vi "Test_API_GetGlobalLogInstance_ValidLogInstanceReturned.vi"(8 "error in (no error)":errorcluster, 11 "TestCase in":refnum<class "TestComposedLog.lvclass">) -> (0 "error out":errorcluster, 3 "TestCase out":refnum<class "TestComposedLog.lvclass">)   [LabVIEW 2017, in "TestComposedLog.lvclass"]
uses:
  TestComposedLog.lvclass
  Source/Composed Log/Types/Log Level.ctl
  Source/Composed Log/LoggerReference/LoggerReference.lvclass/LoggerReference.ctl
  26ac907e-b197-4f92-b50b-edca335a3ee8.vi
  26ac907e-b197-4f92-b50b-edca335a3ee8.vi/98f69271-1de1-4081-8ac1-8b840b0807ac.vi
  Source/Composed Log/Singleton Event Log/Get Nested Global Log Instance.vi/b2f05d58-65df-4e80-8f90-78513ac31376.vi
  Source/Composed Log/LoggerReference/Return Aggregate Queues.vi
  Source/Composed Log/LoggerReference/Add Aggregate Log.vi
  26ac907e-b197-4f92-b50b-edca335a3ee8.vi/98f69271-1de1-4081-8ac1-8b840b0807ac.vi/bbd2f978-e444-4445-9202-4eeb40a61ae4.vi
  Source/Composed Log/Singleton Event Log/Get Nested Global Log Instance.vi/b2f05d58-65df-4e80-8f90-78513ac31376.vi/e1ecde32-be62-4caa-aa7a-1c02d969ae2d.vi
  Source/Composed Log/LoggerReference/Send Add Sink.vi
  Source/LVQueue Sink/LVQueue Sink.lvclass
  C:/CS/Internal/LabVIEW/Logger/Source/Composed Log/Log Sink/Log Sink.lvclass
  Source/Composed Log/Application Logger/Launch Worker Loop.vi
  Source/Composed Log/LoggerReference/Initialize Logger Instance.vi
  Source/Composed Log/Singleton Event Log/Logger Queue FGV.vi
  Source/Composed Log/Singleton Event Log/Shared Instance FGV.vi
  Source/Composed Log/IErrorFormat/IErrorFormat.lvclass
  Source/Composed Log/LoggerReference/LoggerReference.lvclass
  Source/Composed Log/Log Sink/Log Sink.lvclass
  <vilib>/addons/_JKI Toolkits/VI Tester/TestCase.llb/TestCase.lvclass
  Source/Composed Log/Composed Log.lvlib
  Source/Composed Log/Singleton Event Log/Singleton Event Log.lvlib
  C:/Program Files (x86)/National Instruments/LabVIEW 2017/vi.lib/addons/_JKI Toolkits/VI Tester/TestCase.llb/TestCase.lvclass
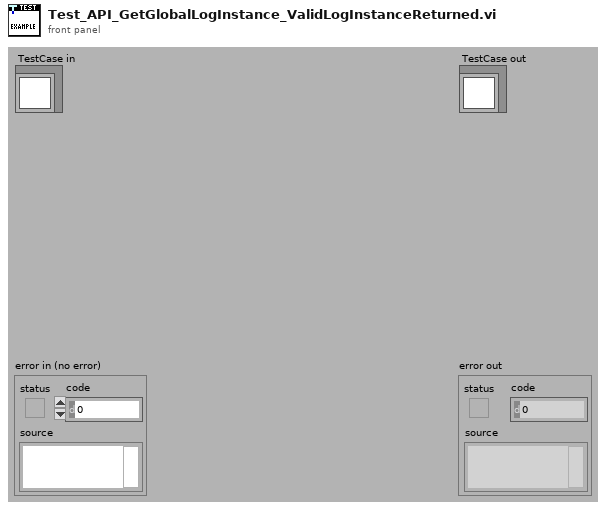
[diagram p1: front panel]
types:
  T1 = typedef "Composed Log.lvlib/Log Level.ctl" = enum16{"Debug", "Info", "Warning", "Error", "Critical"}
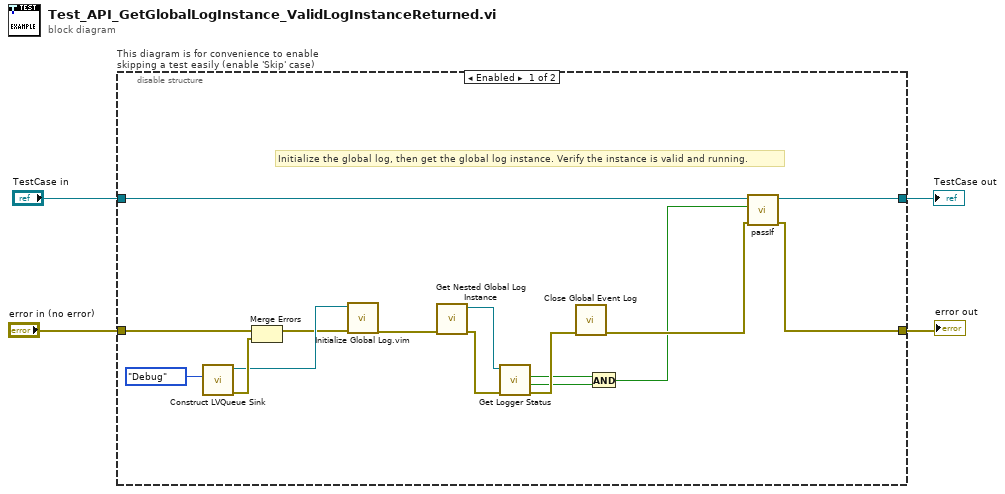
[diagram p0: block diagram]
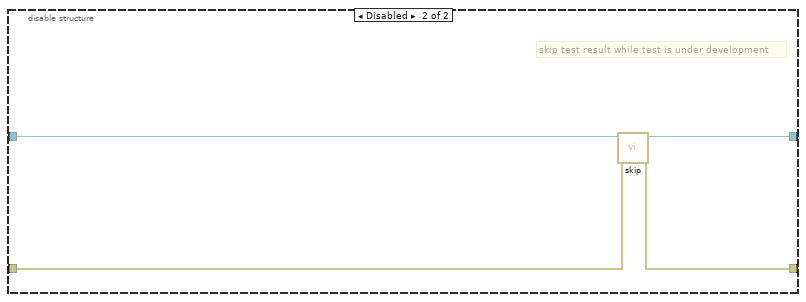
[diagram p2: hidden frame]
diagram:
  n1 = disable-structure "This diagram is for convenience to enable skipping a test easily (enable 'Skip' case)" shown="Enabled" {
    disable-tunnel: "TestCase in" -> [w11 w24]
    disable-tunnel: [w10 w22] -> w1
    disable-tunnel: [w8 w23] -> w3
    disable-tunnel: "error in (no error)" -> [w20 w21]
    frame Enabled {
      # "Initialize the global log, then get the global log instance. Verify the instance is valid and running."
      n2 = call "Construct LVQueue Sink.vi"("LogLevel"=Log_Level."Debug") -> ("error out"=w18:errorcluster, "LVQueue Sink out"=w17:refnum<class "LVQueue Sink.lvclass">)  [unwired: 9 in]
      n3 = Merge Errors(w20, w18) -> (w16:errorcluster)
      n4 = call "Initialize Global Log.vim"("error in (no error)"=w16, "Log Sink(s)"=w17) -> ("error out"=w15:errorcluster)  [unwired: 8 in, 1 out]
      n5 = call "Get Nested Global Log Instance.vi"("error in (no error)"=w15) -> ("error out"=w14:errorcluster, "Nested Global Log Instance Reference"=w13:refnum<class "LoggerReference.lvclass">)  [unwired: 9 in]
      n6 = call "Get Logger Status.vi"("error in (no error)"=w14, "LoggerReference in"=w13) -> ("error out"=w12:errorcluster, "Logger Running?"=w7:bool, "Logger Instantiated?"=w6:bool)  [unwired: 6 in, 1 out]
      n7 = call "Close Global Event Log.vi"("error in (no error)"=w12) -> ("error out"=w9:errorcluster)  [unwired: 10 in]
      n8 = And(x=w6, y=w7) -> (x .and. y?=w5:bool)
      n9 = call-dynamic "passIf.vi"("error in (no error)"=w9, "pass"=w5, "TestCase in"=w11) -> ("error out"=w8:errorcluster, "TestCase out"=w10:refnum<class "TestComposedLog.lvclass">)  [unwired: 7 in]
    }
    frame Disabled {
      # "skip test result while test is under development"
      n10 = call <vilib>:"skip.vi"("error in (no error)"=w21, "TestCase in"=w24) -> ("error out"=w23:errorcluster, "TestCase out"=w22:refnum<class "TestComposedLog.lvclass">)  [unwired: 8 in]
    }
  }
  "error out" <- w3
  "TestCase out" <- w1
